vi "Persist Entity.vi"(8 "error in (no error)":errorcluster, 9 "Entity":refnum<class "Entity.lvclass">, 10 "Types":refnum<class "Type.lvclass">[](array[class]), 11 "SQLite in":refnum<class "SQLite.lvclass">) -> (0 "error out":errorcluster, 3 "SQLite out":refnum<class "SQLite.lvclass">)   [LabVIEW 2020, in "Conditum SQLite.lvlib" / "SQLite.lvclass"]
uses:
  SQLite.lvclass
  SQLite.lvclass/SQLite.ctl
  <vilib>/IlluminatedG/IG Conditum Base/Conditum/Entity/Entity.lvclass
  <vilib>/drjdpowell/SQLite Library/SQL Connection/Connection.lvclass
  <vilib>/drjdpowell/SQLite Library/Transaction Helpers/Transaction.lvlib
  <vilib>/IlluminatedG/IG Conditum Base/Conditum/Columns/Type/Type.lvclass
  <vilib>/IlluminatedG/IG Conditum Base/Conditum/Columns/Boolean/Boolean.lvclass
  <vilib>/IlluminatedG/IG Conditum Base/Conditum/Columns/Integer/Integer.lvclass
  <vilib>/IlluminatedG/IG Conditum Base/Conditum/Columns/Double/Double.lvclass
  <vilib>/IlluminatedG/IG Conditum Base/Conditum/Columns/Timestamp/Timestamp.lvclass
  <vilib>/IlluminatedG/IG Conditum Base/Conditum/Columns/String/String.lvclass
  <vilib>/drjdpowell/SQLite Library/SQL Statement/SQL Statement.lvclass
  <vilib>/IlluminatedG/IG Conditum Base/Conditum/Columns/ID/ID.lvclass
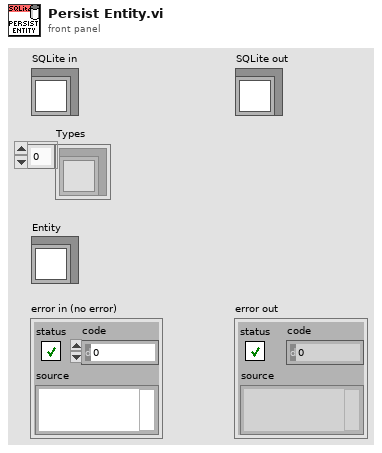
[diagram p1: front panel]
types:
  T1 = typedef "Conditum.lvlib/Field Type.ctl" = enum16{"None", "ID", "Boolean", "Integer", "Double", "Timestamp", "String", "Text", "Entity"}
  T2 = typedef "Conditum.lvlib/Entity ID.ctl" = i64
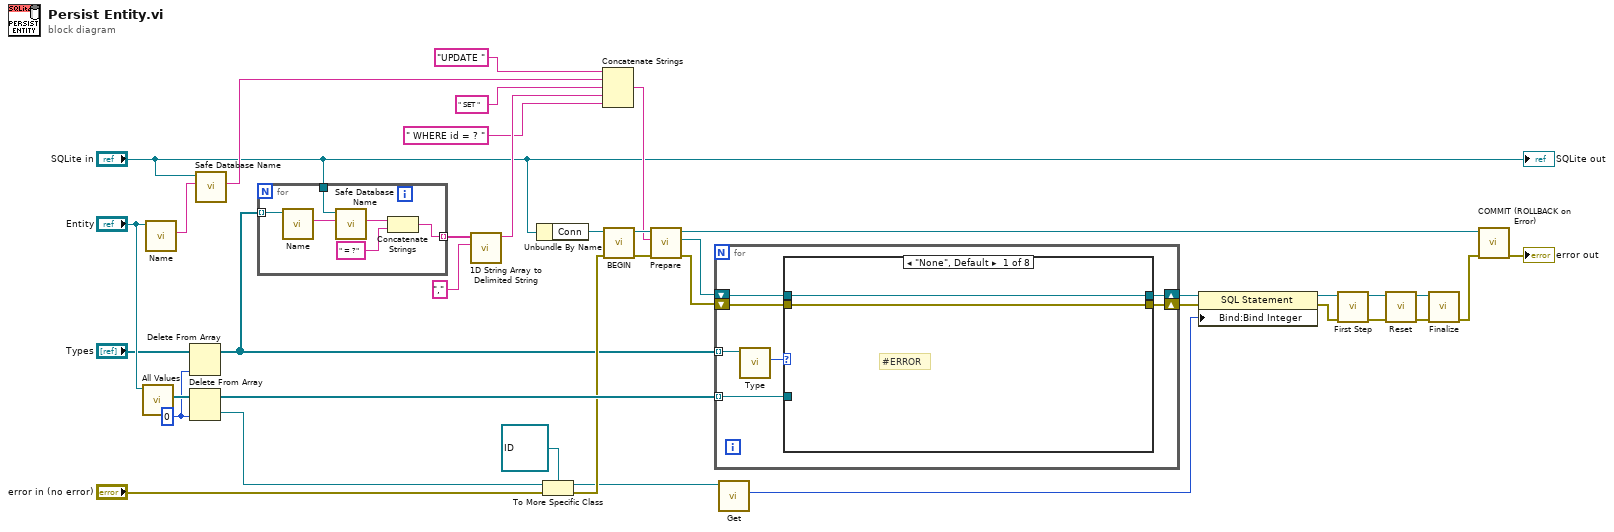
[diagram p0: block diagram]
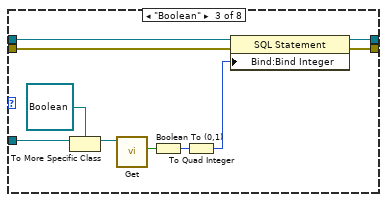
[diagram p3: hidden frame]
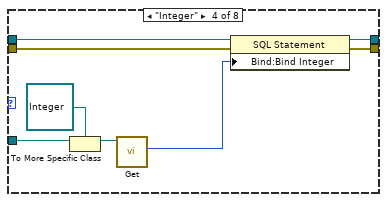
[diagram p4: hidden frame]
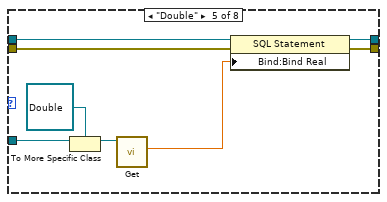
[diagram p5: hidden frame]
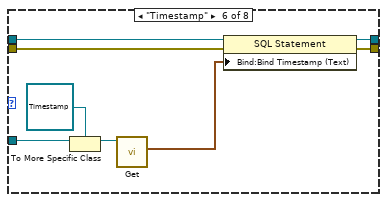
[diagram p6: hidden frame]
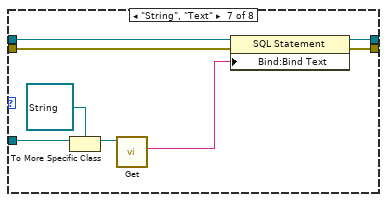
[diagram p7: hidden frame]
diagram:
  w2 = 0 ("index")
  n1 = call <vilib>:"All Values.vi"("Entity in"="Entity") -> ("All Values"=w37:refnum<class "Type.lvclass">[])  [unwired: 10 in]
  n2 = call-dynamic <vilib>:"Name.vi"("Entity in"="Entity") -> ("Name"=w38:string)  [unwired: 10 in]
  n3 = Delete From Array(array="Types", index=w2) -> (array with subset deleted=w1:refnum<class "Type.lvclass">[])  [unwired: 1 in, 1 out]
  n4 = Delete From Array(array=w37, index=w2) -> (deleted portion=w9:refnum<class "Type.lvclass">, array with subset deleted=w23:refnum<class "Type.lvclass">[])  [unwired: 1 in]
  n5 = call-dynamic "Safe Database Name.vi"("Conditum Name"=w38, "Database in"="SQLite in") -> ("Database Name"=w19:string)  [unwired: 9 in]
  n6 = for {
    tunnel: w1 -> [w44] mode=indexing
    tunnel: [w39] -> w22 mode=indexing
    tunnel: "SQLite in" -> [w42]
    n7 = call <vilib>:"Name.vi"("Type in"=w44) -> ("Table Name"=w43:string)  [unwired: 10 in]
    n8 = call-dynamic "Safe Database Name.vi"("Conditum Name"=w43, "Database in"=w42) -> ("Database Name"=w41:string)  [unwired: 9 in]
    n9 = Concatenate Strings(w41, " = ?" ("string")) -> (w39:string)
  }
  n10 = call <vilib>:"1D String Array to Delimited String.vi"("delimiter"=",", "string array"=w22) -> ("delimited string"=w21:string)  [unwired: 9 in]
  n11 = Unbundle By Name("SQLite in") -> ("Conn"=w35:refnum<class "Connection.lvclass">)
  n12 = To More Specific Class(target class=refnum<class "ID.lvclass"> refnum ("Conditum:Columns:ID.lvclass"), reference=w9, error in="error in (no error)") -> (specific class reference=w5:refnum<class "ID.lvclass">, error out=w6:errorcluster)
  n13 = Concatenate Strings("UPDATE ", w19, " SET " ("string"), w21, " WHERE id = ? " ("string")) -> (w32:string)
  n14 = call <vilib>:"BEGIN.vi"("error in (no error)"=w6, "SQLite Connection in"=w35) -> ("error out"=w33:errorcluster, "SQLite Connection"=w34:refnum<class "Connection.lvclass">)  [unwired: 8 in]
  n15 = call <vilib>:"Prepare.vi"("error in (no error)"=w33, "SQL"=w32, "SQLite Connection in"=w34) -> ("error out"=w30:errorcluster, "SQL Statement"=w31:refnum<class "SQL Statement.lvclass">, "SQLite Connection"=w25:refnum<class "Connection.lvclass">)  [unwired: 4 in, 2 out]
  n16 = for {
    shift-right: [w47] -> w13
    shift-left: w31 -> [w51]
    shift-right: [w46] -> w12
    shift-left: w30 -> [w50]
    tunnel: w23 -> [w48] mode=indexing
    tunnel: w1 -> [w45] mode=indexing
    n17 = call <vilib>:"Type.vi"("Type in"=w45) -> ("Type"=w49:T1)  [unwired: 10 in]
    n18 = case shown="\"None\", Default" w49 {
      tunnel: w51 -> [w53 w55 w62 w70 w78 w86 w94 w99]
      tunnel: w50 -> [w52 w54 w58 w69 w77 w85 w93 w98]
      tunnel: w48 -> [_ _ w65 w73 w81 w89 w97 _]
      tunnel: [w53 w55 w57 w68 w76 w84 w92 w99] -> w47
      tunnel: [w52 w54 w56 w67 w75 w83 w91 w98] -> w46
      frame "None", Default {
        # "#ERROR"
      }
      frame "ID" {
        # "#ERROR"
      }
      frame "Boolean" {
        n19 = To More Specific Class(target class=refnum<class "Boolean.lvclass"> refnum ("Conditum:Columns:Boolean.lvclass"), reference=w65) -> (specific class reference=w63:refnum<class "Boolean.lvclass">)  [unwired: 1 in, 1 out]
        n20 = call <vilib>:"Get.vi"("Boolean in"=w63) -> ("Value"=w61:bool)  [unwired: 10 in]
        n21 = Boolean To (0,1)(Boolean=w61) -> (0, 1=w60:i16)
        n22 = To Quad Integer(1:w60) -> (0:w59:i64)
        n23 = property class="SQL Statement"(reference=w62, error in=w58, "Bind:Bind Integer"=w59) -> (reference out=w57:refnum<class "SQL Statement.lvclass">, error out=w56:errorcluster)
      }
      frame "Integer" {
        n24 = To More Specific Class(target class=refnum<class "Integer.lvclass"> refnum ("Conditum:Columns:Integer.lvclass"), reference=w73) -> (specific class reference=w71:refnum<class "Integer.lvclass">)  [unwired: 1 in, 1 out]
        n25 = call <vilib>:"Get.vi"("Integer in"=w71) -> ("Value"=w66:i64)  [unwired: 10 in]
        n26 = property class="SQL Statement"(reference=w70, error in=w69, "Bind:Bind Integer"=w66) -> (reference out=w68:refnum<class "SQL Statement.lvclass">, error out=w67:errorcluster)
      }
      frame "Double" {
        n27 = To More Specific Class(target class=refnum<class "Double.lvclass"> refnum ("Conditum:Columns:Double.lvclass"), reference=w81) -> (specific class reference=w79:refnum<class "Double.lvclass">)  [unwired: 1 in, 1 out]
        n28 = call <vilib>:"Get.vi"("Double in"=w79) -> ("Value"=w74:dbl)  [unwired: 10 in]
        n29 = property class="SQL Statement"(reference=w78, error in=w77, "Bind:Bind Real"=w74) -> (reference out=w76:refnum<class "SQL Statement.lvclass">, error out=w75:errorcluster)
      }
      frame "Timestamp" {
        n30 = To More Specific Class(target class=refnum<class "Timestamp.lvclass"> refnum ("Conditum:Columns:Timestamp.lvclass"), reference=w89) -> (specific class reference=w87:refnum<class "Timestamp.lvclass">)  [unwired: 1 in, 1 out]
        n31 = call <vilib>:"Get.vi"("Timestamp in"=w87) -> ("Value"=w82:timestamp)  [unwired: 10 in]
        n32 = property class="SQL Statement"(reference=w86, error in=w85, "Bind:Bind Timestamp (Text)"=w82) -> (reference out=w84:refnum<class "SQL Statement.lvclass">, error out=w83:errorcluster)
      }
      frame "String", "Text" {
        n33 = To More Specific Class(target class=refnum<class "String.lvclass"> refnum ("Conditum:Columns:String.lvclass"), reference=w97) -> (specific class reference=w95:refnum<class "String.lvclass">)  [unwired: 1 in, 1 out]
        n34 = call <vilib>:"Get.vi"("String in"=w95) -> ("Value"=w90:string)  [unwired: 10 in]
        n35 = property class="SQL Statement"(reference=w94, error in=w93, "Bind:Bind Text"=w90) -> (reference out=w92:refnum<class "SQL Statement.lvclass">, error out=w91:errorcluster)
      }
      frame "Entity" {
        # "#TODO\nRelation update"
      }
    }
  }
  n36 = call <vilib>:"Get.vi"("ID in"=w5) -> ("Entity ID"=w4:T2)  [unwired: 10 in]
  n37 = property class="SQL Statement"(reference=w13, error in=w12, "Bind:Bind Integer"=w4) -> (reference out=w11:refnum<class "SQL Statement.lvclass">, error out=w10:errorcluster)
  n38 = call <vilib>:"First Step.vi"("error in (no error)"=w10, "SQL Statement in"=w11) -> ("error out"=w29:errorcluster, "SQL Statement"=w28:refnum<class "SQL Statement.lvclass">)  [unwired: 7 in, 1 out]
  n39 = call <vilib>:"Reset.vi"("error in (no error)"=w29, "SQL Statement in"=w28) -> ("error out"=w27:errorcluster, "SQL Statement"=w26:refnum<class "SQL Statement.lvclass">)  [unwired: 8 in]
  n40 = call <vilib>:"Finalize.vi"("error in (no error)"=w27, "SQL Statement in"=w26) -> ("error out"=w24:errorcluster)  [unwired: 9 in]
  n41 = call <vilib>:"COMMIT (ROLLBACK on Error).vi"("error in (no error)"=w24, "SQLite Connection in"=w25) -> ("error out"=→"error out":errorcluster)  [unwired: 8 in, 1 out]
  "SQLite out" <- "SQLite in"
